vi "Do Scope Action.vi"(8 "error in (no error)":errorcluster, 9 "Action Data In":variant, 10 "Scope Action":T1, 11 "Actor_Scope in":refnum<class "Actor_Scope.lvclass">) -> (0 "error out":errorcluster, 3 "Actor_Scope out":refnum<class "Actor_Scope.lvclass">)   [LabVIEW 2020, in "Actor_Scope.lvlib" / "Actor_Scope.lvclass"]
uses:
  Actor_Scope.lvclass
  Scope_Action.ctl
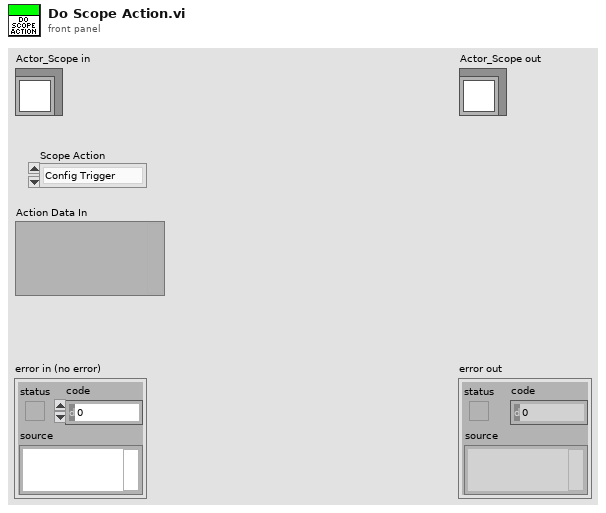
[diagram p1: front panel]
types:
  T1 = typedef "Actor_Scope.lvlib/Actor_Scope.lvclass/Scope_Action.ctl" = enum16{"Config Trigger", "Init Wfm Acq", "Read Wfm"}
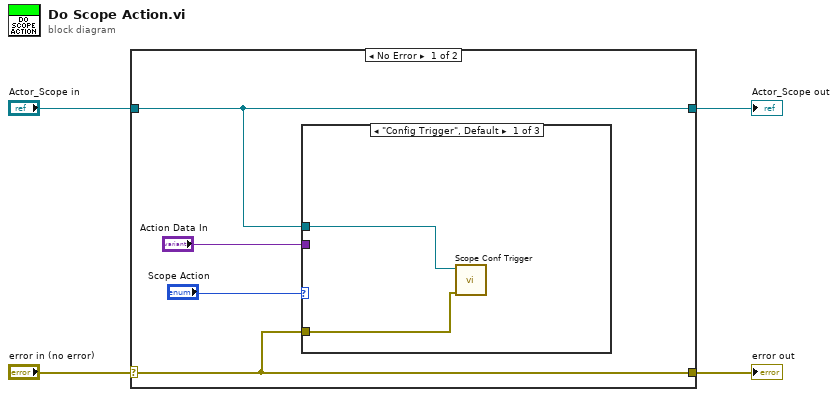
[diagram p0: block diagram]
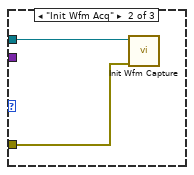
[diagram p2: hidden frame]
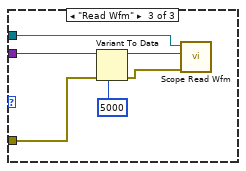
[diagram p3: hidden frame]
diagram:
  n1 = case shown="No Error" "error in (no error)" {
    selector: "error in (no error)" -> [w7 w20]
    tunnel: [w7 w20] -> w3
    tunnel: [w8 w19] -> w1
    tunnel: "Actor_Scope in" -> [w8 w19]
    frame No Error {
      n2 = case shown="\"Config Trigger\", Default" "Scope Action" {
        tunnel: w8 -> [w10 w12 w16]
        tunnel: w7 -> [w9 w11 w14]
        tunnel: "Action Data In" -> [_ _ w18]
        frame "Config Trigger", Default {
          n3 = call-dynamic "Scope Conf Trigger.vi"("error in (no error)"=w9, "Actor_Scope in"=w10) -> ()  [unwired: 8 in, 2 out]
        }
        frame "Init Wfm Acq" {
          n4 = call-dynamic "Init Wfm Capture.vi"("error in (no error)"=w11, "Actor_Scope in"=w12) -> ()  [unwired: 8 in, 2 out]
        }
        frame "Read Wfm" {
          n5 = Variant To Data(error in=w14, type=u32 5000 ("TimeOut"), Variant=w18) -> (data=w15:u32, error out=w13:errorcluster)
          n6 = call-dynamic "Scope Read Wfm.vi"("error in (no error)"=w13, "TimeOut"=w15, "Actor_Scope in"=w16) -> ()  [unwired: 7 in, 2 out]
        }
      }
    }
    frame Error {
    }
  }
  "error out" <- w3
  "Actor_Scope out" <- w1
